vi "Create Event Timing Measurement Tree Layout.vi"(8 "error in (no error)":errorcluster, 9 "window":string, 10 "measurement name":string, 11 "Section Ptr":T1 format="%.0x") -> (0 "error out":errorcluster, 3 "Section Ptr dup":T1 format="%.0x")   [LabVIEW 2020, in "Engine Simulation Toolkit System Explorer.lvlib"]
uses:
  Engine Simulation Toolkit System Explorer.lvlib
  <vilib>/NI VeriStand/Custom Device API/Custom Device Item Ref.ctl
  <vilib>/NI VeriStand/Custom Device API/Custom Device Channel Type.ctl
  Shared/Constants and GUIDs.vi
  Shared/Properties.vi
  <vilib>/NI VeriStand/Custom Device API/Set Item Property (String).vi
  <vilib>/NI VeriStand/Custom Device API/Custom Device API.lvlib
  Shared/Engine Simulation Toolkit Shared.lvlib
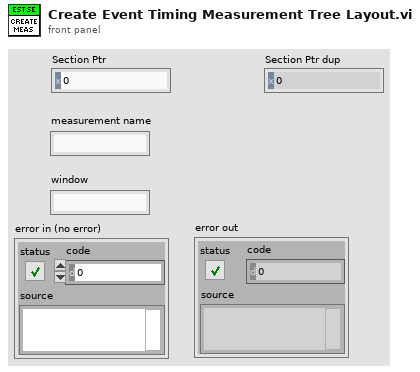
[diagram p1: front panel]
types:
  T1 = typedef "Custom Device API.lvlib/Custom Device Item Ref.ctl" = u64
  T2 = typedef "Custom Device API.lvlib/Custom Device Channel Type.ctl" = enum16{"Input", "Output"}
  T3 = typedef "Engine Simulation Toolkit Shared.lvlib/Channel.ctl" = cluster{"Name":string, "Units":string, "Default":dbl, "Description":string, "Scalable":bool}
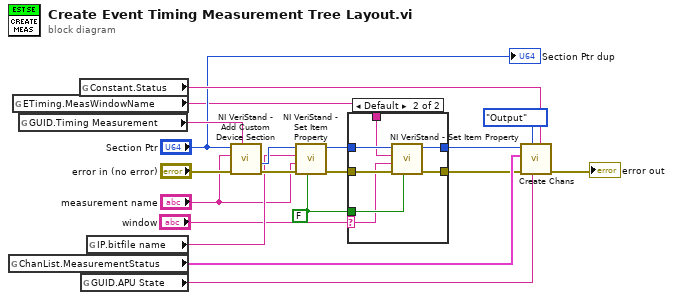
[diagram p0: block diagram]
diagram:
  w2 = FALSE ("Binary String (T)")
  n1 = global read "Constants and GUIDs.vi" "ChanList.MeasurementStatus"() -> (w14:T3[])
  n2 = global read "Properties.vi" "ETiming.MeasWindowName"() -> (w3:string)
  n3 = global read "Constants and GUIDs.vi" "GUID.Timing Measurement"() -> (w18:string)
  n4 = global read "Constants and GUIDs.vi" "Constant.Status"() -> (w15:string)
  n5 = global read "Constants and GUIDs.vi" "GUID.APU State"() -> (w12:string)
  n6 = global read "Properties.vi" "IP.bitfile name"() -> (w9:string)
  n7 = call <vilib>:"NI VeriStand - Add Custom Device Section.vi"("GUID (Default Section)"=w18, "error in (no error)"="error in (no error)", "Section Name"="measurement name", "Parent Ref in"="Section Ptr") -> ("error out"=w17:errorcluster, "Section Ptr"=w10:T1)  [unwired: 4 in, 2 out]
  n8 = call-poly <vilib>:"NI VeriStand - Set Item Property.vi"("Binary String (T)"=w2, "error in (no error)"=w17, "Value"="measurement name", "Property Name"=w9, "Item Ref in"=w10) -> ("error out"=w11:errorcluster, "Item Ref out"=w5:T1)  [unwired: 4 in, 1 out]
  n9 = case shown="Default" "window" {
    selector: "window" -> [_ w22]
    tunnel: w11 -> [w20 w28]
    tunnel: [w20 w27] -> w6
    tunnel: w5 -> [w21 w26]
    tunnel: [w21 w25] -> w4
    tunnel: w3 -> [_ w24]
    tunnel: w2 -> [_ w23]
    frame "" {
    }
    frame Default {
      n10 = call-poly <vilib>:"NI VeriStand - Set Item Property.vi"("Binary String (T)"=w23, "error in (no error)"=w28, "Value"=w22, "Property Name"=w24, "Item Ref in"=w26) -> ("error out"=w27:errorcluster, "Item Ref out"=w25:T1)  [unwired: 4 in, 1 out]
    }
  }
  n11 = call "Create Chans.vi"("New Section Name (none)"=w15, "new section GUID (\"\":del prot)"=w12, "Type"=Custom_Device_Channel_Type."Output", "error in (no error)"=w6, "Channels"=w14, "Section Ptr"=w4) -> ("error out"=→"error out":errorcluster)  [unwired: 2 in, 3 out]
  "Section Ptr dup" <- "Section Ptr"
